vi "Rename LVClass.vi"(7 "App reference":refnum<vi>, 8 "error in (no error)":errorcluster, 10 "Destination Path":path, 11 "Source Class Path":path) -> (0 "error out":errorcluster, 3 "Updated LVClass Path":path)   [LabVIEW 2011, in "VITesterUtilities.lvlib"]
uses:
  Libraries/VITesterUtilities.lvlib
  <userlib>/_OpenG.lib/file/file.llb/Strip Path Extension - Path__ogtk.vi
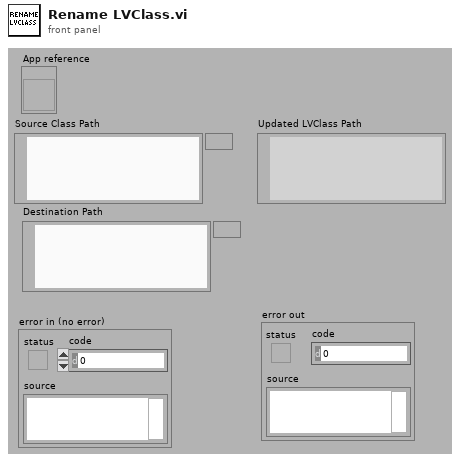
[diagram p1: front panel]
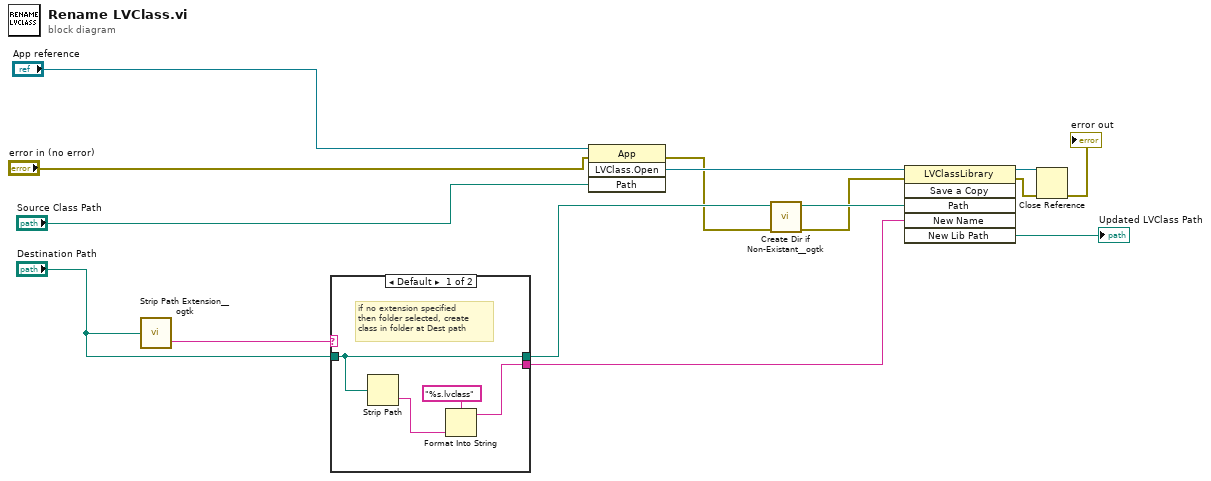
[diagram p0: block diagram]
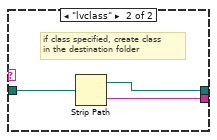
[diagram p2: hidden frame]
diagram:
  n1 = call-poly <userlib>:"Strip Path Extension__ogtk.vi"("path"="Destination Path") -> ("extension"=w5:string)  [unwired: 1 out]
  n2 = case shown="Default" w5 {
    tunnel: [w17 w22] -> w7
    tunnel: [w16 w20] -> w4
    tunnel: "Destination Path" -> [w16 w21]
    frame Default {
      # "if no extension specified\nthen folder selected, create\nclass in folder at Dest path"
      n3 = Strip Path(path=w16) -> (name=w19:string)  [unwired: 1 out]
      n4 = Format Into String(format string="%s.lvclass", w19) -> (resulting string=w17:string)  [unwired: 2 in, 1 out]
    }
    frame "lvclass" {
      # "if class specified, create class\nin the destination folder"
      n5 = Strip Path(path=w21) -> (stripped path=w20:path, name=w22:string)
    }
  }
  n6 = invoke class="App" method="LVClass.Open"(reference="App reference", error in="error in (no error)", "Path"="Source Class Path") -> (error out=w2:errorcluster, "LVClass.Open"=w14:refnum<vi>)  [unwired: 1 in, 2 out]
  n7 = call <userlib>:"Create Dir if Non-Existant__ogtk.vi"("error in (no error)"=w2, "Directory Path"=w4) -> ("error out"=w1:errorcluster, "dup Directory Path"=w3:path)  [unwired: 7 in, 1 out]
  n8 = invoke class="LVClassLibrary" method="Save a Copy"(reference=w14, error in=w1, "Path"=w3, "New Name"=w7) -> (reference out=w13:refnum<vi>, error out=w12:errorcluster, "New Lib Path"=→"Updated LVClass Path":path)  [unwired: 2 in, 3 out]
  n9 = Close Reference(reference=w13, error in (no error)=w12) -> (error out=→"error out":errorcluster)
